vi "StupidGlobal.vi"() -> ()   [LabVIEW 2014, in "Elevator System.lvlib"]
uses:
  Elevator System.lvlib
panel:
  out "Cycle2":bool
  in  "Enum":enum16{"Down", "Up", "Auto"}(ring)=enum."Auto"
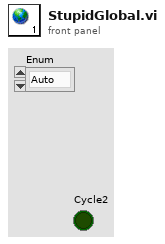
[diagram p1: front panel]
diagram:
